vi "Calibrate Light Array.vi"() -> ()   [LabVIEW 2016]
panel:
  out "index":i32=25
  in  "Index":cluster{"Numeric":i32}[][](array[cluster])=[[{"Numeric"=3}, {"Numeric"=9}, {"Numeric"=2}, {"Numeric"=8}, {"Numeric"=19}, {"Numeric"=23}], [{"Numeric"=1}, {"Numeric"=11}, {"Numeric"=0}, {"Numeric"=10}, {"Numeric"=17}, {"Numeric"=21}], [{"Numeric"=5}, {"Numeric"=-1}, {"Numeric"=4}, {"Numeric"=14}, {"Numeric"=27}, {"Numeric"=25}], [{"Numeric"=7}, {"Numeric"=13}, {"Numeric"=6}, {"Numeric"=12}, {"Numeric"=26}, {"Numeric"=24}], [{"Numeric"=29}, {"Numeric"=31}, {"Numeric"=-1}, {"Numeric"=18}, {"Numeric"=-1}, {"Numeric"=22}], [{"Numeric"=30}, {"Numeric"=16}, {"Numeric"=-1}, {"Numeric"=-1}, {"Numeric"=-1}, {"Numeric"=-1}]]
  out "Light Array Index":i32=31
  out "Calibration":i32[](array[numeric])=[8, 6, 2, 0, 14, 12, 20, 18, 3, 1, 9, 7, 21, 19, 15, 19, 31, 10, 27, 4, 31, 11, 29, 5, 23, 17, 22, 16, 29, 24, 30, 25]
  in  "physical channels":refnum<k21>="Dev0/Ao0:15"
  in  "physical channels 2":refnum<k21>="Dev1/Ao0:15"
  out "log2(x)":i32=25
  in  "Light Array":cluster{"Boolean":bool}[][](array[cluster])=[[{"Boolean"=FALSE}, {"Boolean"=FALSE}, {"Boolean"=FALSE}, {"Boolean"=FALSE}, {"Boolean"=FALSE}, {"Boolean"=FALSE}], [{"Boolean"=FALSE}, {"Boolean"=FALSE}, {"Boolean"=FALSE}, {"Boolean"=FALSE}, {"Boolean"=FALSE}, {"Boolean"=FALSE}], [{"Boolean"=FALSE}, {"Boolean"=FALSE}, {"Boolean"=FALSE}, {"Boolean"=FALSE}, {"Boolean"=FALSE}, {"Boolean"=FALSE}], [{"Boolean"=FALSE}, {"Boolean"=FALSE}, {"Boolean"=FALSE}, {"Boolean"=FALSE}, {"Boolean"=FALSE}, {"Boolean"=FALSE}], [{"Boolean"=FALSE}, {"Boolean"=FALSE}, {"Boolean"=FALSE}, {"Boolean"=FALSE}, {"Boolean"=FALSE}, {"Boolean"=FALSE}], [{"Boolean"=FALSE}, {"Boolean"=FALSE}, {"Boolean"=FALSE}, {"Boolean"=FALSE}, {"Boolean"=FALSE}, {"Boolean"=FALSE}]]
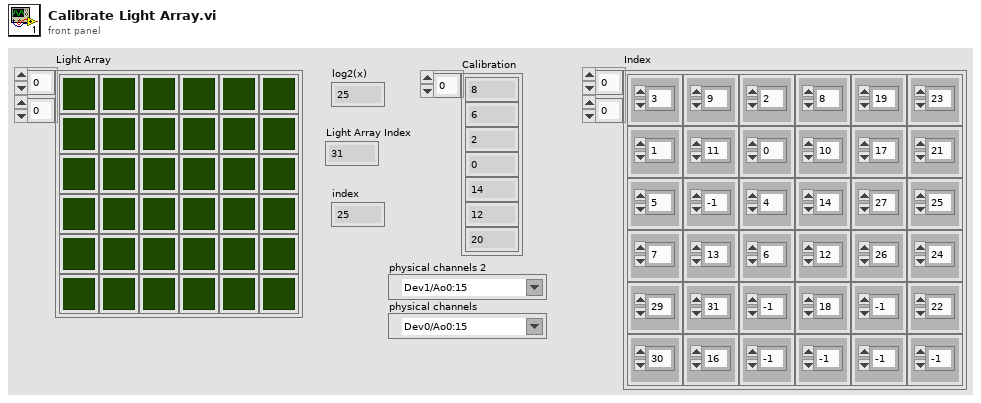
[diagram p1: front panel]
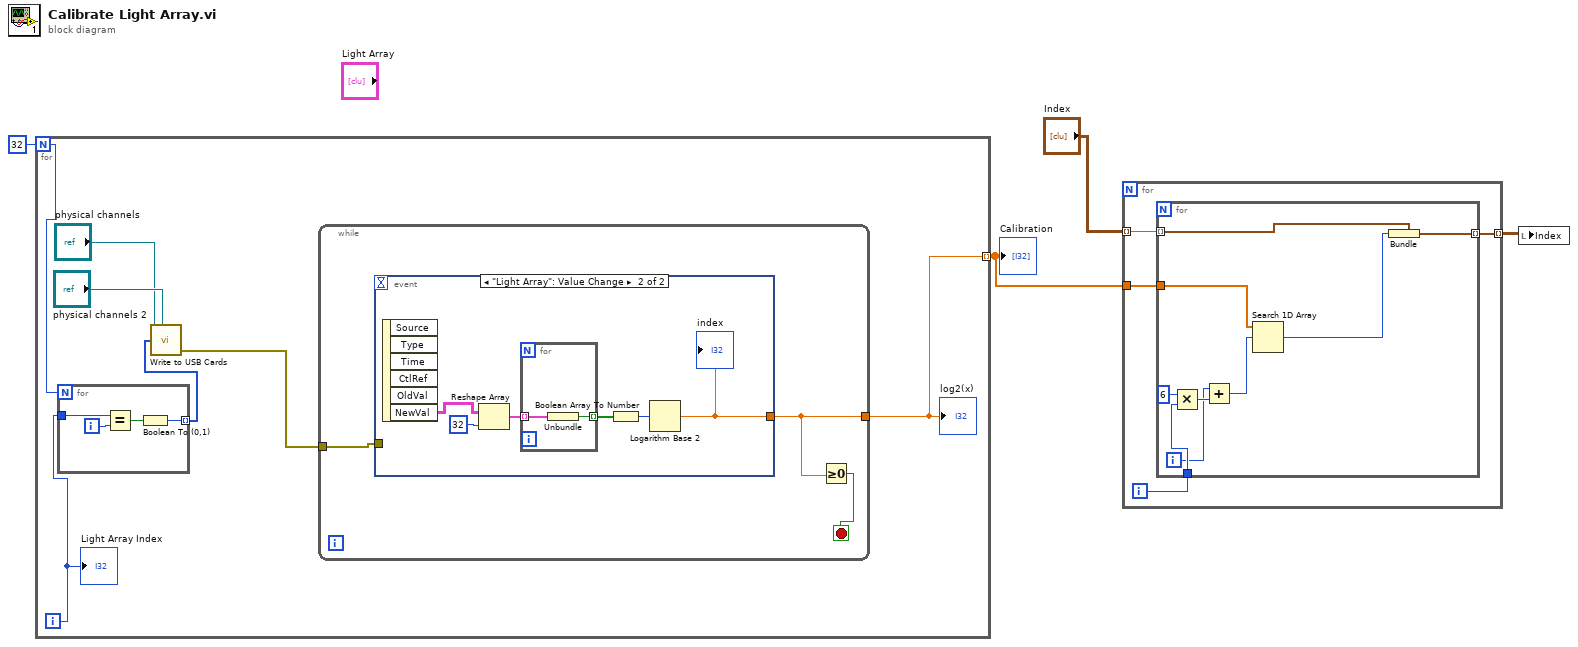
[diagram p0: block diagram]
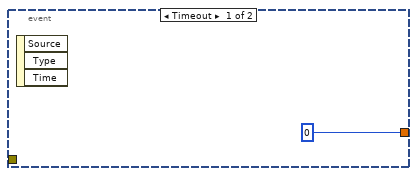
[diagram p2: hidden frame]
diagram:
  n1 = for {
    N: 32 -> [w5]
    tunnel: [w6] -> w2 mode=indexing
    i -> [w9]
    n2 = for {
      N: w5 -> [_]
      tunnel: w9 -> [w26]
      tunnel: [w24] -> w8 mode=indexing
      i -> [w27]
      n3 = Equal?(x=w26, y=w27) -> (x = y?=w25:bool)
      n4 = Boolean To (0,1)(Boolean=w25) -> (0, 1=w24:i16)
    }
    n5 = call "Write to USB Cards.vi"("physical channels"="physical channels", "physical channels 2"="physical channels 2", "Array"=w8) -> ("error out"=w7:errorcluster)  [unwired: 6 in]
    n6 = while {
      tunnel: w7 -> [w14]
      tunnel: [w13] -> w6
      stop <- w12 stop-if-true
      n7 = event shown="[1] \"Light Array\": Value Change" {
        selector: _ -> [_ _]
        dyn-events: _ -> [_ _]
        timeout: _ -> [_ _]
        tunnel: [u32 0 w16] -> w13
        tunnel: w14 -> [_ _]
        event Timeout {
          n8 = event-data() -> ()  [unwired: 1 in, 3 out]
        }
        event "Light Array": Value Change {
          n9 = event-data() -> ("NewVal"=w17:cluster{"Boolean":bool}[][])  [unwired: 1 in, 5 out]
          n10 = Reshape Array(w17, 32 ("dimension size")) -> (w20:cluster{"Boolean":bool}[])
          n11 = for {
            tunnel: w20 -> [w23] mode=indexing
            tunnel: [w22] -> w18 mode=indexing
            n12 = Unbundle(w23) -> ("Boolean"=w22:bool)
          }
          n13 = Boolean Array To Number(Boolean array=w18) -> (number=w19:u32)
          n14 = Logarithm Base 2(1:w19) -> (0:w16:dbl)
          "index" <- w16
        }
      }
      n15 = Greater Or Equal To 0?(x=w13) -> (x >= 0?=w12:bool)
    }
    "log2(x)" <- w6
    "Light Array Index" <- w9
  }
  "Calibration" <- w2
  n16 = for {
    tunnel: "Index" -> [w31] mode=indexing
    tunnel: w2 -> [w29]
    tunnel: [w28] -> w1 mode=indexing
    i -> [w30]
    n17 = for {
      tunnel: w31 -> [w33] mode=indexing
      tunnel: w30 -> [w40]
      tunnel: w29 -> [w36]
      tunnel: [w32] -> w28 mode=indexing
      i -> [w37]
      n18 = Multiply(x=6, y=w40) -> (x*y=w38:i32)
      n19 = Add(x=w37, y=w38) -> (x+y=w35:i32)
      n20 = Search 1D Array(1D array=w36, element=w35) -> (index of element=w34:i32)  [unwired: 1 in]
      n21 = Bundle(cluster=w33, "Numeric"=w34) -> (w32:cluster{"Numeric":i32})
    }
  }
  n22 = local write "Index"(w1) -> ()
